vi "RP Lockin Sweeper.vi"(6 "Samples per read":i32=1024, 8 "Error In":errorcluster, 9 "Dwell time":dbl=0.01, 10 "Frequencies":dbl[](array[numeric]), 11 "connection ID":refnum<k5>) -> (0 "Error Out":errorcluster, 1 "Y":dbl[](array[numeric]), 2 "X":dbl[](array[numeric]), 3 "connection ID out":refnum<k5>)   [LabVIEW 2015]
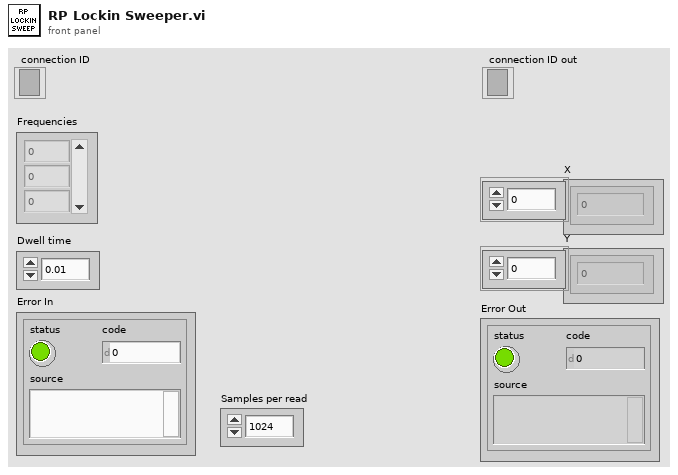
[diagram p1: front panel]
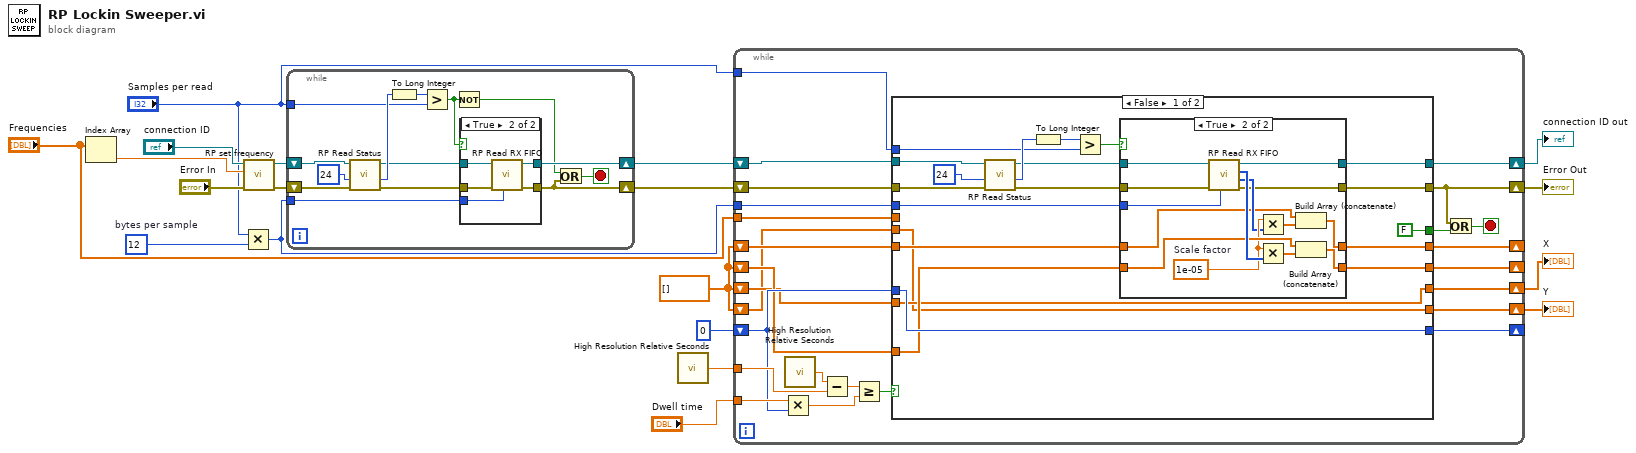
[diagram p0: block diagram]
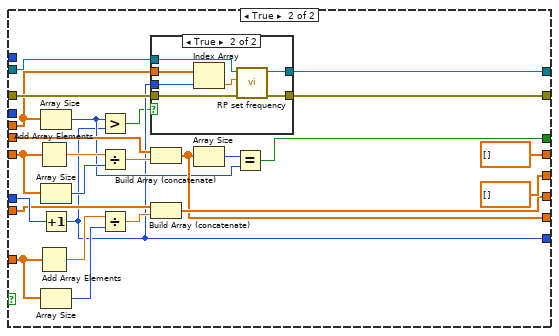
[diagram p4: hidden frame]
diagram:
  w11 = dbl[] [] ("x*y")
  w12 = 12  # bytes per sample
  n1 = Index Array(array="Frequencies") -> (element=w16:dbl)  [unwired: 1 in]
  n2 = Multiply(x="Samples per read", y=w12) -> (x*y=w1:i32)
  n3 = call "RP set frequency.vi"("Error In"="Error In", "Frequency"=w16, "connection ID"="connection ID") -> ("Error Out"=w2:errorcluster, "connection ID out"=w5:refnum<k5>)  [unwired: 6 in, 1 out]
  n4 = while {
    tunnel: "Samples per read" -> [w30]
    shift-right: [w20] -> w3
    shift-left: w2 -> [w27]
    shift-right: [w25] -> w4
    shift-left: w5 -> [w26]
    tunnel: w1 -> [w24]
    stop <- w23 stop-if-true
    n5 = call "RP Read Status.vi"("Error In"=w27, "Status offset"=u64 24, "connection ID"=w26) -> ("Error Out"=w22:errorcluster, "Status response"=w31:u32, "connection ID out"=w29:refnum<k5>)  [unwired: 6 in]
    n6 = To Long Integer(number=w31) -> (32bit integer=w32:i32)
    n7 = Greater?(x=w32, y=w30) -> (0:w28:bool)
    n8 = Not(x=w28) -> (.not. x?=w21:bool)
    n9 = case shown="True" w28 {
      tunnel: w29 -> [w35 w40]
      tunnel: w22 -> [w34 w39]
      tunnel: [w34 w38] -> w20
      tunnel: [w35 w37] -> w25
      tunnel: w24 -> [_ w36]
      frame False {
      }
      frame True {
        n10 = call "RP Read RX FIFO.vi"("FIFO Bytes per read"=w36, "Error In"=w39, "connection ID"=w40) -> ("Error Out"=w38:errorcluster, "connection ID out"=w37:refnum<k5>)  [unwired: 4 in, 3 out]
      }
    }
    n11 = Or(x=w21, y=w20) -> (x .or. y?=w23:bool)
  }
  n12 = call <vilib>:"High Resolution Relative Seconds.vi"() -> ("relative seconds"=w17:dbl)
  n13 = while {
    shift-right: [w57] -> _
    shift-left: 0 -> [w59]
    tunnel: "Dwell time" -> [w65]
    tunnel: w17 -> [w61]
    tunnel: "Frequencies" -> [w58]
    shift-right: [w54] -> _
    shift-left: w11 -> [w53]
    shift-right: [w51] -> _
    shift-left: w11 -> [w52]
    tunnel: "Samples per read" -> [w56]
    tunnel: w1 -> [w55]
    shift-right: [w47] -> w10
    shift-left: w11 -> [w50]
    shift-right: [w48] -> w9
    shift-left: w11 -> [w49]
    shift-right: [w41] -> w7
    shift-left: w3 -> [w46]
    shift-right: [w44] -> w8
    shift-left: w4 -> [w45]
    stop <- w42 stop-if-true
    n14 = Multiply(x=w65, y=w59) -> (x*y=w64:dbl)
    n15 = call <vilib>:"High Resolution Relative Seconds.vi"() -> ("relative seconds"=w63:dbl)
    n16 = Subtract(x=w63, y=w61) -> (x-y=w62:dbl)
    n17 = Greater Or Equal?(x=w62, y=w64) -> (x >= y?=w60:bool)
    n18 = case shown="False" w60 {
      tunnel: w59 -> [w85 w120]
      tunnel: w58 -> [_ w110]
      tunnel: [w85 w105] -> w57
      tunnel: w56 -> [w82 _]
      tunnel: w55 -> [w81 _]
      tunnel: [w77 dbl[] [] ("x*y")] -> w54
      tunnel: w53 -> [w76 w126]
      tunnel: w52 -> [w75 w121]
      tunnel: [w74 dbl[] [] ("x*y")] -> w51
      tunnel: w50 -> [w73 w119]
      tunnel: w49 -> [w72 w117]
      tunnel: [w72 w109] -> w48
      tunnel: [w73 w115] -> w47
      tunnel: w46 -> [w71 w114]
      tunnel: [w69 w113] -> w41
      tunnel: w45 -> [w68 w112]
      tunnel: [w67 w111] -> w44
      tunnel: [FALSE w107] -> w43
      frame False {
        n19 = call "RP Read Status.vi"("Error In"=w71, "Status offset"=u64 24, "connection ID"=w68) -> ("Error Out"=w70:errorcluster, "Status response"=w83:u32, "connection ID out"=w78:refnum<k5>)  [unwired: 6 in]
        n20 = To Long Integer(number=w83) -> (32bit integer=w80:i32)
        n21 = Greater?(x=w80, y=w82) -> (0:w79:bool)
        n22 = case shown="True" w79 {
          tunnel: w81 -> [_ w103]
          tunnel: w78 -> [w86 w102]
          tunnel: [w89 w100] -> w77
          tunnel: w76 -> [w89 w98]
          tunnel: w75 -> [w88 w94]
          tunnel: [w88 w93] -> w74
          tunnel: w70 -> [w87 w92]
          tunnel: [w87 w91] -> w69
          tunnel: [w86 w90] -> w67
          frame False {
          }
          frame True {
            w97 = 1e-05  # Scale factor
            n23 = call "RP Read RX FIFO.vi"("FIFO Bytes per read"=w103, "Error In"=w92, "connection ID"=w102) -> ("Error Out"=w91:errorcluster, "Y"=w96:i32[], "X"=w101:i32[], "connection ID out"=w90:refnum<k5>)  [unwired: 4 in, 1 out]
            n24 = Multiply(x=w97, y=w96) -> (x*y=w95:dbl[])
            n25 = Multiply(x=w97, y=w101) -> (x*y=w99:dbl[])
            n26 = Build Array (concatenate)(w94, w95) -> (w93:dbl[])
            n27 = Build Array (concatenate)(w98, w99) -> (w100:dbl[])
          }
        }
      }
      frame True {
        n28 = Add Array Elements(numeric array=w121) -> (sum=w122:dbl)
        n29 = Add Array Elements(numeric array=w126) -> (sum=w125:dbl)
        n30 = Array Size(array=w110) -> (size(s)=w106:i32)
        n31 = Array Size(array=w121) -> (size(s)=w123:i32)
        n32 = Increment(x=w120) -> (x+1=w105:i32)
        n33 = Array Size(array=w126) -> (size(s)=w124:i32)
        n34 = Greater?(x=w106, y=w105) -> (0:w104:bool)
        n35 = Divide(x=w122, y=w123) -> (x/y=w116:dbl)
        n36 = Divide(x=w125, y=w124) -> (x/y=w118:dbl)
        n37 = case shown="True" w104 {
          tunnel: w105 -> [_ w136]
          tunnel: w114 -> [w129 w135]
          tunnel: [w129 w134] -> w113
          tunnel: w112 -> [w130 w133]
          tunnel: [w130 w132] -> w111
          tunnel: w110 -> [_ w131]
          frame False {
          }
          frame True {
            n38 = Index Array(array=w131, index=w136) -> (element=w137:dbl)
            n39 = call "RP set frequency.vi"("Error In"=w135, "Frequency"=w137, "connection ID"=w133) -> ("Error Out"=w134:errorcluster, "connection ID out"=w132:refnum<k5>)  [unwired: 6 in, 1 out]
          }
        }
        n40 = Build Array (concatenate)(w117, w116) -> (w109:dbl[])
        n41 = Build Array (concatenate)(w119, w118) -> (w115:dbl[])
        n42 = Array Size(array=w109) -> (size(s)=w108:i32)
        n43 = Equal?(x=w108, y=w106) -> (x = y?=w107:bool)
      }
    }
    n44 = Or(x=w41, y=w43) -> (x .or. y?=w42:bool)
  }
  "connection ID out" <- w8
  "X" <- w10
  "Y" <- w9
  "Error Out" <- w7
